vi "CIF Manager UI.vi"() -> ()   [LabVIEW 2021, in "CIF Manager UI.lvlib"]
uses:
  CIF Manager UI.lvlib
  CIFUI/Typedef/CIF_Manager_UI_Tab.ctl
  CIFUI/Typedef/Subpanel Type.ctl
  CIFUI/Typedef/Core UI References.ctl
  CIFUI/CIF_UI.lvclass/CIF_UI.ctl
  CIFUI/Utilities/Get Human Readable Error.vi
  <vilib>/CIF Foundation/CIF Utilities/Errors/Append Error Location.vi
  CIFUI/UI Element Update/Empty Tree by Reference.vi
  CIFUI/UI Element Update/Empty Table by Reference.vi
  CIFUI/UI Element Update/Initialize Manager Tab by Reference.vi
  <vilib>/CIF Foundation/CIF Utilities/Errors/Human Readable Error Message.vi
  CIFUI/CIF_UI.lvclass
panel:
  in  "Clear Local Error":bool
  out "System Errors":bool
  in  "EXIT":bool
  in  "Address":string="192.168.1.160"
  out "Connected":bool
  in  "Connection":bool
  in  "CIF Manager UI Tab":T1
  out "Local Error":string
  in  "Session Id":u64
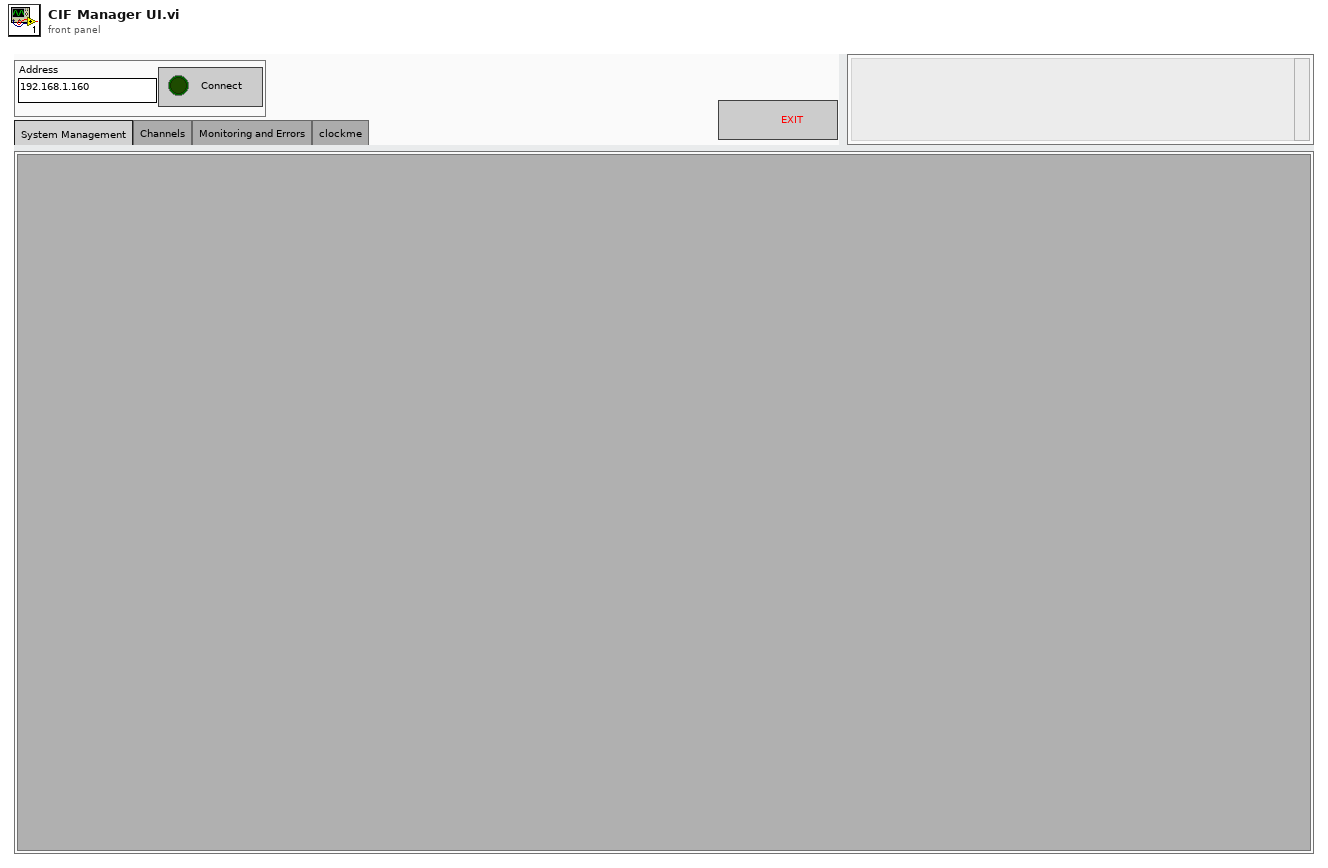
[diagram p1: front panel]
types:
  T1 = typedef "CIF_UI.lvclass/CIF_Manager_UI_Tab.ctl" = enum32{"System Management", "Channels", "Monitoring and Errors", "Plugin UI"}
  T2 = typedef "CIF_UI.lvclass/Subpanel Type.ctl" = enum16{"System", "Errors", "Channel", "Plugin"}
  T3 = typedef "CIF_UI.lvclass/Core UI References.ctl" = cluster{"Discovered Plugins":refnum<vi>, "Discovered Plugins Valid":bool, "Loaded Plugins":refnum<vi>, "Loaded Plugins Valid":bool, "Publisher Channels":refnum<vi>, "Publisher Channels Valid":bool, "Subscriber Channels":refnum<vi>, "Subscriber Channels Valid":bool, "Plugin Status":refnum<vi>, "Plugin Status Valid":bool, "Channel Connection":refnum<vi>, "Channel Connection Valid":bool, "New Plugin Load":refnum<vi>, "New Plugin Load Valid":bool, "Errors":refnum<vi>, "Errors Valid":bool, "Plugin to Abort":refnum<vi>, "Plugin to Abort Valid":bool, "Connection":refnum<vi>, "Connection Valid":bool, "Exit":refnum<vi>, "Exit Valid":bool, "Run Listen":refnum<vi>, "Run Listen Valid":bool, "CIF Manager Tab":refnum<vi>, "Manger Tab Valid":bool, "Clear Local Error":refnum<vi>, "Clear Local Error Valid":bool, "Local Error":refnum<vi>, "Local Error Valid":bool, "System Errors":refnum<vi>, "System Errors Valid":bool, "Plugin Selection":refnum<vi>, "Plugin Selection Valid":bool}
  T4 = typedef "CIF_InstrumentStudio Plugin SDK.lvlib/Event Registration Refnum.ctl" = refnum<event-registration>
  T5 = cluster{"Event Refnum":T4, "Event Registration Refnum":refnum<event-registration>}
  T6 = typedef "CIF_Manager_UI_Tab.ctl" = enum32{"System Management", "Channels", "Monitoring and Errors", "Plugin UI"}
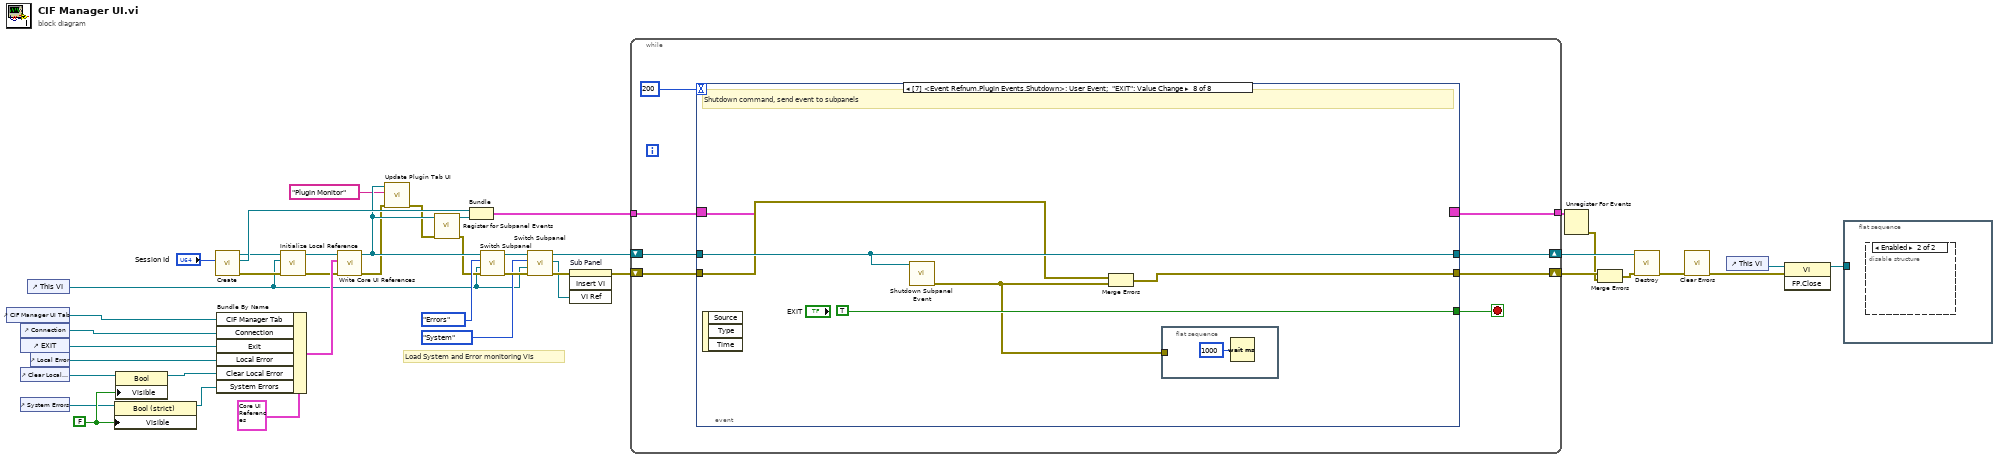
[diagram p0: block diagram]
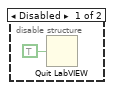
[diagram p2: hidden frame]
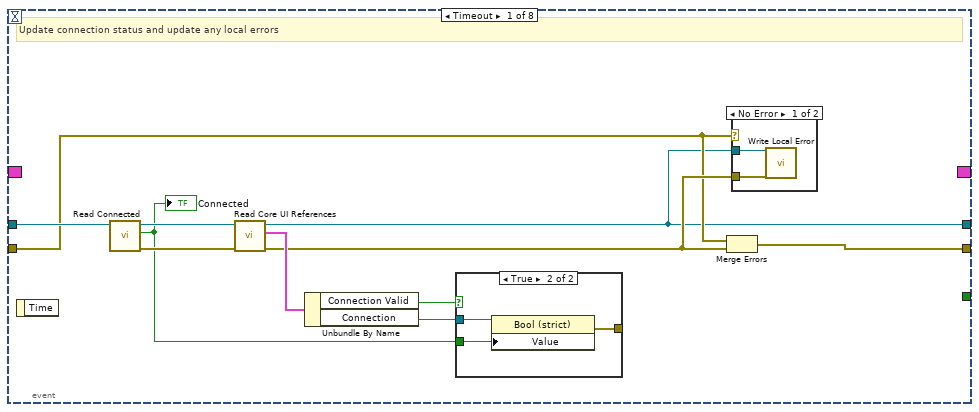
[diagram p3: hidden frame]
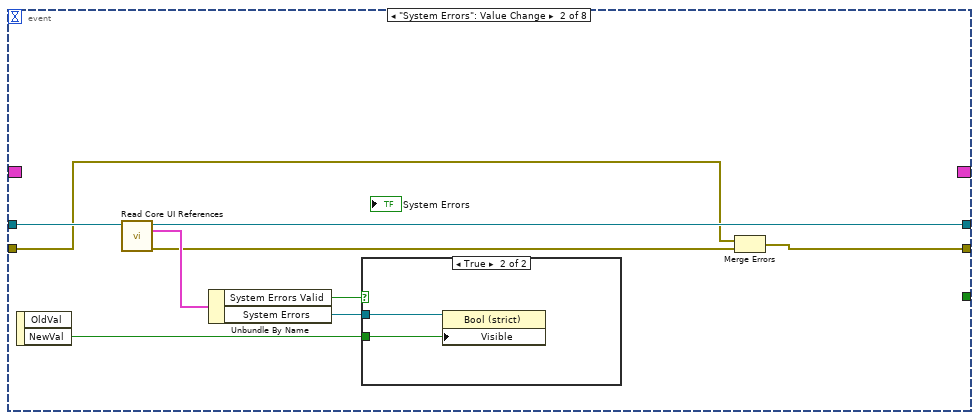
[diagram p6: hidden frame]
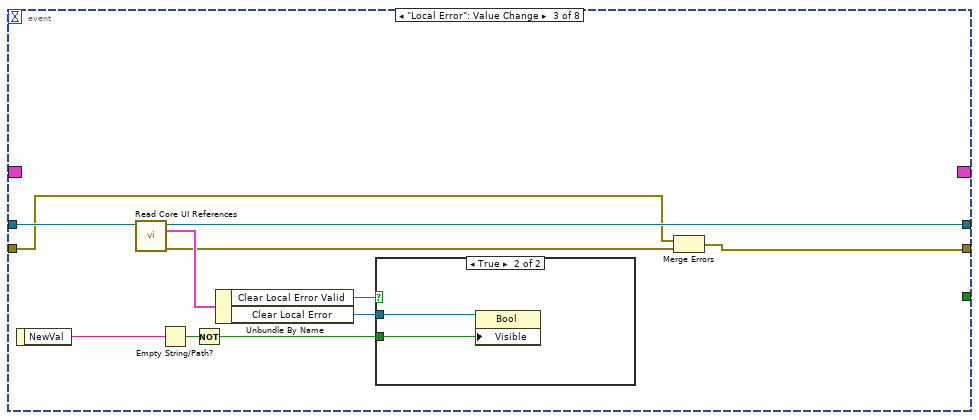
[diagram p8: hidden frame]
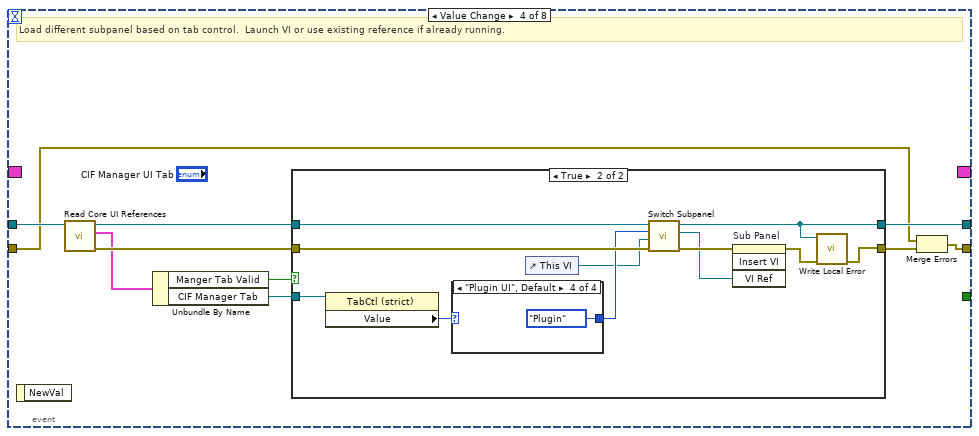
[diagram p10: hidden frame]
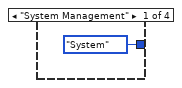
[diagram p12: hidden frame]
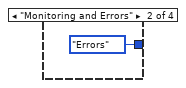
[diagram p13: hidden frame]
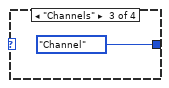
[diagram p14: hidden frame]
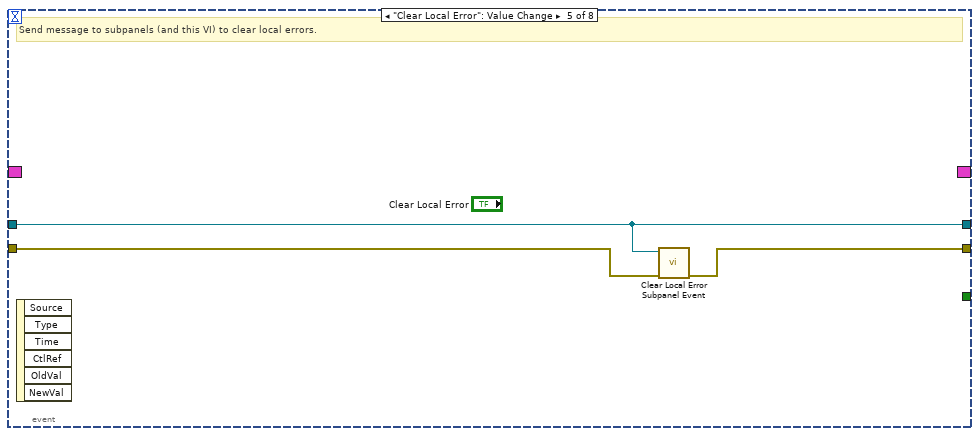
[diagram p15: hidden frame]
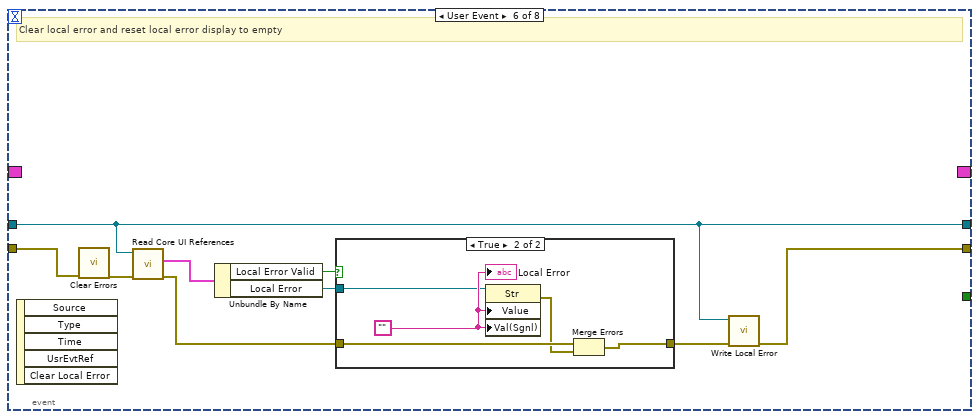
[diagram p16: hidden frame]
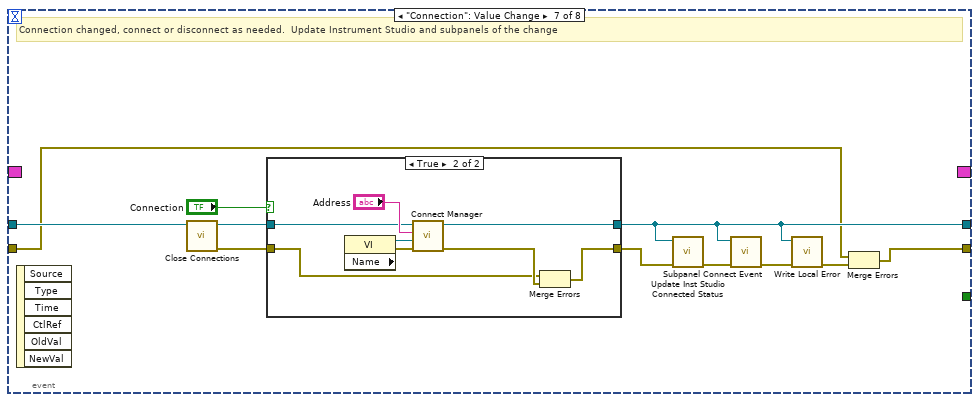
[diagram p18: hidden frame]
diagram:
  w10 = FALSE ("Visible")
  # "Load System and Error monitoring VIs"
  n1 = control-ref of="CIF Manager UI Tab"() -> (w36:refnum<vi>)
  n2 = control-ref of="Connection"() -> (w37:refnum<vi>)
  n3 = control-ref of="EXIT"() -> (w38:refnum<vi>)
  n4 = control-ref of="Clear Local Error"() -> (w13:refnum<vi>)
  n5 = control-ref of="System Errors"() -> (w9:refnum<vi>)
  n6 = control-ref of="This VI"() -> (w8:refnum<vi>)
  n7 = control-ref of="Local Error"() -> (w12:refnum<vi>)
  n8 = property class="Bool (strict)"(reference=w9, "Visible"=w10) -> (reference out=w14:refnum<vi>)  [unwired: 1 in, 1 out]
  n9 = property class="Bool"(reference=w13, "Visible"=w10) -> (reference out=w11:refnum<vi>)  [unwired: 1 in, 1 out]
  n10 = call "Create.vi"("Session Id"="Session Id") -> ("error out"=w23:errorcluster, "Event Refnum"=w34:T4, "CIF_UI out"=w24:refnum<class "CIF_UI.lvclass">)  [unwired: 8 in]
  n11 = Bundle By Name(cluster=T3 {"Discovered Plugins"=refnum, "Discovered Plugins Valid"=FALSE, "Loaded Plugins"=refnum, "Loaded Plugins Valid"=FALSE, "Publisher Channels"=refnum, "Publisher Channels Valid"=FALSE, "Subscriber Channels"=refnum, "Subscriber Channels Valid"=FALSE, "Plugin Status"=refnum, "Plugin Status Valid"=FALSE, "Channel Connection"=refnum, "Channel Connection Valid"=FALSE, "New Plugin Load"=refnum, "New Plugin Load Valid"=FALSE, "Errors"=refnum, "Errors Valid"=FALSE, "Plugin to Abort"=refnum, "Plugin to Abort Valid"=FALSE, "Connection"=refnum, "Connection Valid"=FALSE, "Exit"=refnum, "Exit Valid"=FALSE, "Run Listen"=refnum, "Run Listen Valid"=FALSE, "CIF Manager Tab"=refnum, "Manger Tab Valid"=FALSE, "Clear Local Error"=refnum, "Clear Local Error Valid"=FALSE, "Local Error"=refnum, "Local Error Valid"=FALSE, "System Errors"=refnum, "System Errors Valid"=FALSE, "Plugin Selection"=refnum, "Plugin Selection Valid"=FALSE} ("UI References"), "CIF Manager Tab"=w36, "Connection"=w37, "Exit"=w38, "Local Error"=w12, "Clear Local Error"=w11, "System Errors"=w14) -> (w39:T3)
  n12 = call "Initialize Local Reference.vi"("error in (no error)"=w23, "This VI"=w8, "CIF_UI in"=w24) -> ("error out"=w22:errorcluster, "CIF_UI out"=w21:refnum<class "CIF_UI.lvclass">)  [unwired: 7 in]
  n13 = call "Write Core UI References.vi"("error in (no error)"=w22, "UI References"=w39, "CIF_UI in"=w21) -> ("error out"=w16:errorcluster, "CIF_UI out"=w19:refnum<class "CIF_UI.lvclass">)  [unwired: 7 in]
  n14 = call "Update Plugin Tab UI.vi"("error in (no error)"=w16, "Plugin Name"="Plugin Monitor", "CIF_UI in"=w19) -> ("error out"=w17:errorcluster)  [unwired: 8 in]
  n15 = call "Register for Subpanel Events.vi"("error in (no error)"=w17, "CIF_UI in"=w19) -> ("error out"=w18:errorcluster, "Event Registration Refnum"=w35:refnum<event-registration>)  [unwired: 8 in]
  n16 = Bundle("Event Refnum"=w34, "Event Registration Refnum"=w35) -> (w33:T5)  [unwired: 1 in]
  n17 = call "Switch Subpanel.vi"("error in (no error)"=w18, "Calling VI"=w8, "Subpanel Type"=Subpanel_Type."Errors", "CIF_UI in"=w19) -> ("error out"=w27:errorcluster, "CIF_UI out"=w28:refnum<class "CIF_UI.lvclass">)  [unwired: 5 in, 1 out]
  n18 = call "Switch Subpanel.vi"("error in (no error)"=w27, "Calling VI"=w8, "Subpanel Type"=Subpanel_Type."System", "CIF_UI in"=w28) -> ("error out"=w31:errorcluster, "VI Reference"=w29:refnum<vi>, "CIF_UI out"=w32:refnum<class "CIF_UI.lvclass">)  [unwired: 5 in]
  n19 = invoke on="Sub Panel" class="SubPnl" method="Insert VI"(error in=w31, "VI Ref"=w29) -> (error out=w30:errorcluster)  [unwired: 2 in, 3 out]
  n20 = while {
    shift-right: [w46] -> w42
    shift-left: w32 -> [w48]
    shift-right: [w43] -> w5
    shift-left: w30 -> [w47]
    tunnel: w33 -> [w45]
    tunnel: [w44] -> w20
    stop <- w49 stop-if-true
    n21 = event shown="[7] <Event Refnum.Plugin Events.Shutdown>: User Event;  \"EXIT\": Value Change" {
      selector: w45 -> [_ _ _ _ _ _ _ _]
      dyn-events: [_ _ _ _ _ _ _ _] -> w44
      timeout: 200 -> [_ _ _ _ _ _ _ _]
      tunnel: [_ _ _ _ _ _ _ TRUE] -> w49
      tunnel: w48 -> [w61 w75 w85 w99 w120 w121 w146 w160]
      tunnel: w47 -> [w53 w69 w79 w91 w119 w128 w137 w159]
      tunnel: [w51 w67 w78 w92 w118 w122 w136 w158] -> w43
      tunnel: [w52 w74 w84 w100 w120 w121 w139 w160] -> w46
      event Timeout {
        # "Update connection status and update any local errors"
        n22 = event-data() -> ()  [unwired: 1 in, 1 out]
        n23 = call "Read Connected.vi"("CIF_UI in"=w61) -> ("error out"=w59:errorcluster, "Connected"=w55:bool, "CIF_UI out"=w60:refnum<class "CIF_UI.lvclass">)  [unwired: 8 in]
        "Connected" <- w55
        n24 = call "Read Core UI References.vi"("error in (no error)"=w59, "CIF_UI in"=w60) -> ("error out"=w54:errorcluster, "UI References"=w56:T3, "CIF_UI out"=w52:refnum<class "CIF_UI.lvclass">)  [unwired: 7 in]
        n25 = Unbundle By Name(w56) -> ("Connection Valid"=w58:bool, "Connection"=w57:refnum<vi>)
        n26 = case shown="True" w58 {
          tunnel: w57 -> [_ w66]
          tunnel: w55 -> [_ w65]
          tunnel: [_ w64] -> _
          frame False {
          }
          frame True {
            n27 = property class="Bool (strict)"(reference=w66, "Value"=w65) -> (error out=w64:errorcluster)  [unwired: 1 in, 1 out]
          }
        }
        n28 = Merge Errors(w53, w54) -> (w51:errorcluster)
        n29 = case shown="No Error" w53 {
          tunnel: w52 -> [w63 _]
          tunnel: w54 -> [w62 _]
          frame No Error {
            n30 = call "Write Local Error.vi"("error in (no error)"=w62, "CIF_UI in"=w63) -> ()  [unwired: 9 in, 1 out]
          }
          frame Error {
          }
        }
      }
      event "System Errors": Value Change {
        n31 = event-data() -> ("NewVal"=w70:bool)  [unwired: 1 in, 1 out]
        n32 = call "Read Core UI References.vi"("CIF_UI in"=w75) -> ("error out"=w68:errorcluster, "UI References"=w73:T3, "CIF_UI out"=w74:refnum<class "CIF_UI.lvclass">)  [unwired: 8 in]
        n33 = Unbundle By Name(w73) -> ("System Errors Valid"=w72:bool, "System Errors"=w71:refnum<vi>)
        n34 = case shown="True" w72 {
          tunnel: w71 -> [_ w77]
          tunnel: w70 -> [_ w76]
          frame False {
          }
          frame True {
            n35 = property class="Bool (strict)"(reference=w77, "Visible"=w76) -> ()  [unwired: 1 in, 2 out]
          }
        }
        n36 = Merge Errors(w69, w68) -> (w67:errorcluster)
      }
      event "Local Error": Value Change {
        n37 = event-data() -> ("NewVal"=w83:string)  [unwired: 1 in]
        n38 = call "Read Core UI References.vi"("CIF_UI in"=w85) -> ("error out"=w80:errorcluster, "UI References"=w88:T3, "CIF_UI out"=w84:refnum<class "CIF_UI.lvclass">)  [unwired: 8 in]
        n39 = Empty String/Path?(string/path=w83) -> (empty?=w82:bool)
        n40 = Not(x=w82) -> (.not. x?=w81:bool)
        n41 = Unbundle By Name(w88) -> ("Clear Local Error Valid"=w87:bool, "Clear Local Error"=w86:refnum<vi>)
        n42 = case shown="True" w87 {
          tunnel: w86 -> [_ w90]
          tunnel: w81 -> [_ w89]
          frame False {
          }
          frame True {
            n43 = property class="Bool"(reference=w90, "Visible"=w89) -> ()  [unwired: 1 in, 2 out]
          }
        }
        n44 = Merge Errors(w79, w80) -> (w78:errorcluster)
      }
      event Value Change {
        # "Load different subpanel based on tab control.  Launch VI or use existing reference if already running."
        n45 = event-data() -> ()  [unwired: 1 in, 1 out]
        n46 = call "Read Core UI References.vi"("CIF_UI in"=w99) -> ("error out"=w97:errorcluster, "UI References"=w96:T3, "CIF_UI out"=w98:refnum<class "CIF_UI.lvclass">)  [unwired: 8 in]
        n47 = Unbundle By Name(w96) -> ("Manger Tab Valid"=w94:bool, "CIF Manager Tab"=w95:refnum<vi>)
        n48 = case shown="True" w94 {
          tunnel: [w102 w105] -> w100
          tunnel: [w101 w103] -> w93
          tunnel: w98 -> [w102 w111]
          tunnel: w97 -> [w101 w110]
          tunnel: w95 -> [_ w109]
          frame False {
          }
          frame True {
            n49 = property class="TabCtl (strict)"(reference=w109) -> ("Value"=w108:T6)  [unwired: 1 in, 2 out]
            n50 = case shown="\"Plugin UI\", Default" w108 {
              tunnel: [Subpanel_Type."System" ("Subpanel Type") Subpanel_Type."Errors" ("Subpanel Type") Subpanel_Type."Channel" ("Subpanel Type") Subpanel_Type."Plugin" ("Subpanel Type")] -> w107
              frame "System Management" {
              }
              frame "Monitoring and Errors" {
              }
              frame "Channels" {
              }
              frame "Plugin UI", Default {
              }
            }
            n51 = control-ref of="This VI"() -> (w106:refnum<vi>)
            n52 = call "Switch Subpanel.vi"("error in (no error)"=w110, "Calling VI"=w106, "Subpanel Type"=w107, "CIF_UI in"=w111) -> ("error out"=w113:errorcluster, "VI Reference"=w112:refnum<vi>, "CIF_UI out"=w105:refnum<class "CIF_UI.lvclass">)  [unwired: 5 in]
            n53 = invoke on="Sub Panel" class="SubPnl" method="Insert VI"(error in=w113, "VI Ref"=w112) -> (error out=w104:errorcluster)  [unwired: 2 in, 3 out]
            n54 = call "Write Local Error.vi"("error in (no error)"=w104, "CIF_UI in"=w105) -> ("error out"=w103:errorcluster)  [unwired: 9 in]
          }
        }
        n55 = Merge Errors(w91, w93) -> (w92:errorcluster)
      }
      event "Clear Local Error": Value Change {
        # "Send message to subpanels (and this VI) to clear local errors."
        n56 = event-data() -> ()  [unwired: 1 in, 6 out]
        n57 = call "Clear Local Error Subpanel Event.vi"("error in (no error)"=w119, "CIF_UI in"=w120) -> ("error out"=w118:errorcluster)  [unwired: 9 in]
      }
      event User Event {
        # "Clear local error and reset local error display to empty"
        n58 = event-data() -> ()  [unwired: 1 in, 5 out]
        n59 = call <vilib>:"Clear Errors.vi"("error in (no error)"=w128) -> ("error out"=w129:errorcluster)  [unwired: 5 in, 1 out]
        n60 = call "Read Core UI References.vi"("error in (no error)"=w129, "CIF_UI in"=w121) -> ("error out"=w126:errorcluster, "UI References"=w127:T3)  [unwired: 7 in, 1 out]
        n61 = Unbundle By Name(w127) -> ("Local Error Valid"=w125:bool, "Local Error"=w124:refnum<vi>)
        n62 = case shown="True" w125 {
          tunnel: w124 -> [_ w131]
          tunnel: w126 -> [w130 w135]
          tunnel: [w130 w133] -> w123
          frame False {
          }
          frame True {
            w132 = ""
            n63 = property class="Str"(reference=w131, "Value"=w132, "Val(Sgnl)"=w132) -> (error out=w134:errorcluster)  [unwired: 1 in, 1 out]
            n64 = Merge Errors(w135, w134) -> (w133:errorcluster)
            "Local Error" <- w132
          }
        }
        n65 = call "Write Local Error.vi"("error in (no error)"=w123, "CIF_UI in"=w121) -> ("error out"=w122:errorcluster)  [unwired: 9 in]
      }
      event "Connection": Value Change {
        # "Connection changed, connect or disconnect as needed.  Update Instrument Studio and subpanels of the change"
        n66 = event-data() -> ()  [unwired: 1 in, 6 out]
        n67 = call "Close Connections.vi"("CIF_UI in"=w146) -> ("error out"=w145:errorcluster, "CIF_UI out"=w144:refnum<class "CIF_UI.lvclass">)  [unwired: 9 in]
        n68 = case shown="True" "Connection" {
          tunnel: [w148 w152] -> w139
          tunnel: [w147 w151] -> w141
          tunnel: w145 -> [w147 w150]
          tunnel: w144 -> [w148 w149]
          frame False {
          }
          frame True {
            n69 = property class="VI" props=["Name"]() -> (reference out=w156:refnum<vi>, error out=w155:errorcluster)  [unwired: 2 in, 1 out]
            n70 = call "Connect Manager.vi"("error in (no error)"=w155, "VI Reference"=w156, "Address"="Address", "CIF_UI in"=w149) -> ("error out"=w153:errorcluster, "CIF_UI out"=w152:refnum<class "CIF_UI.lvclass">)  [unwired: 6 in]
            n71 = Merge Errors(w150, w153) -> (w151:errorcluster)
          }
        }
        n72 = call "Update Inst Studio Connected Status.vi"("error in (no error)"=w141, "CIF_UI in"=w139) -> ("error out"=w142:errorcluster)  [unwired: 9 in]
        n73 = call "Subpanel Connect Event.vi"("error in (no error)"=w142, "CIF_UI in"=w139) -> ("error out"=w140:errorcluster)  [unwired: 9 in]
        n74 = call "Write Local Error.vi"("error in (no error)"=w140, "CIF_UI in"=w139) -> ("error out"=w138:errorcluster)  [unwired: 9 in]
        n75 = Merge Errors(w137, w138) -> (w136:errorcluster)
      }
      event User Event; "EXIT": Value Change {
        # "Shutdown command, send event to subpanels"
        n76 = event-data() -> ()  [unwired: 1 in, 3 out]
        n77 = call "Shutdown Subpanel Event.vi"("CIF_UI in"=w160) -> ("error out"=w157:errorcluster)  [unwired: 10 in]
        n78 = Merge Errors(w159, w157) -> (w158:errorcluster)
        n79 = flat-sequence {
          tunnel: w157 -> [_]
          frame #0 {
            n80 = Wait (ms)(milliseconds to wait=u32 1000) -> ()  [unwired: 1 out]
          }
        }
      }
    }
  }
  n81 = Unregister For Events(event registration refnum=w20) -> (error out=w4:errorcluster)  [unwired: 1 in]
  n82 = Merge Errors(w5, w4) -> (w3:errorcluster)
  n83 = call "Destroy.vi"("error in (no error)"=w3, "CIF_UI in"=w42) -> ("error out"=w7:errorcluster)  [unwired: 8 in, 1 out]
  n84 = call <vilib>:"Clear Errors.vi"("error in (no error)"=w7) -> ("error out"=w6:errorcluster)  [unwired: 5 in, 1 out]
  n85 = control-ref of="This VI"() -> (w2:refnum<vi>)
  n86 = invoke class="VI" method="FP.Close"(reference=w2, error in=w6) -> (reference out=w1:refnum<vi>)  [unwired: 1 in, 2 out]
  n87 = flat-sequence {
    tunnel: w1 -> [_]
    frame #0 {
      n88 = disable-structure shown="Enabled" {
        frame Disabled {
          n89 = Quit LabVIEW(quit? (T)=TRUE) -> ()
        }
        frame Enabled {
        }
      }
    }
  }
